vi "Synchronizator_DSBSC.vi"(8 "Czestotliwosc_probkowania":dbl, 9 "Czas":dbl, 10 "Czestotliwosc_sygnalu_nosnego":dbl, 11 "Sygnal_zmodulowany":dbl[](array[numeric])) -> (3 "Przesuniecie_fazowe":dbl)   [LabVIEW 2020]
doc: "VI zwraca przesuniecie fazowe, o ktore nalezy skorygowac generowany sygnal nosny."
uses:
  Kontrolki/Parametry_cosinusa.ctl
  <vilib>/Analysis/3filter.llb/Butterworth Filter (DBL).vi
  <vilib>/Analysis/NI_AALBase.lvlib
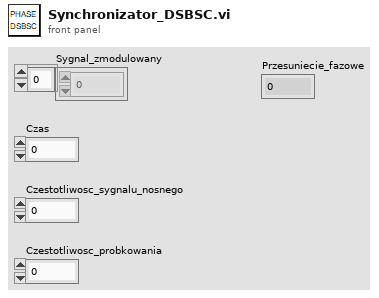
[diagram p1: front panel]
types:
  T1 = typedef "Parametry_cosinusa.ctl" = cluster{"Amplituda [V]":dbl, "Czestotliwosc [Hz] ":dbl, "Faza [rad]":dbl}
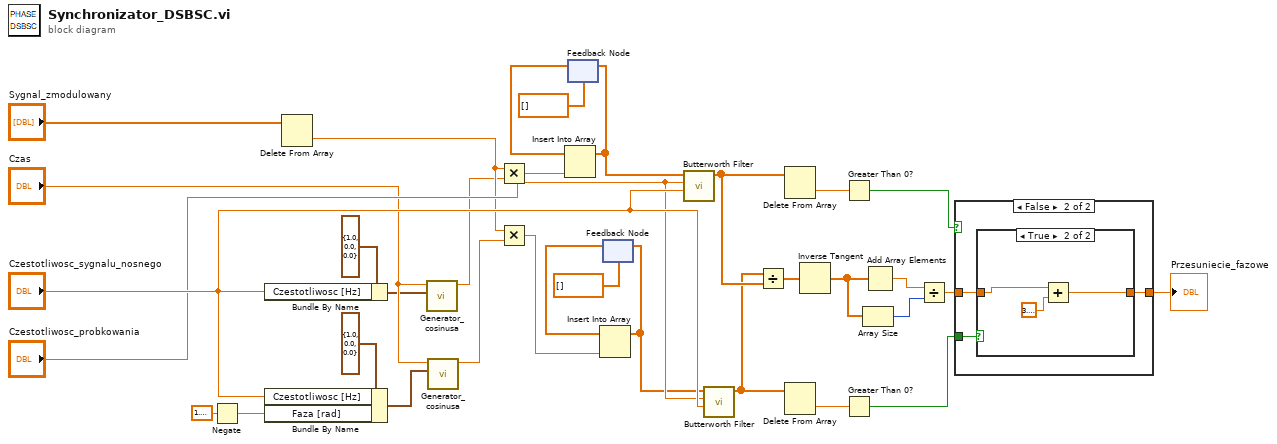
[diagram p0: block diagram]
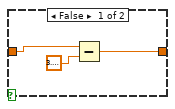
[diagram p4: hidden frame]
diagram:
  n1 = Negate(x=1.5707963267948966) -> (-x=w15:dbl)
  n2 = Bundle By Name(cluster=T1 {"Amplituda [V]"=1.0, "Czestotliwosc [Hz] "=0.0, "Faza [rad]"=0.0} ("Parametry_sygnalu_nosnego"), "Czestotliwosc [Hz]"="Czestotliwosc_sygnalu_nosnego") -> (w11:T1)
  n3 = Bundle By Name(cluster=T1 {"Amplituda [V]"=1.0, "Czestotliwosc [Hz] "=0.0, "Faza [rad]"=0.0} ("Parametry_sygnalu_nosnego"), "Czestotliwosc [Hz]"="Czestotliwosc_sygnalu_nosnego", "Faza [rad]"=w15) -> (w16:T1)
  n4 = Delete From Array(array="Sygnal_zmodulowany") -> (deleted portion=w19:dbl)  [unwired: 2 in, 1 out]
  n5 = call "Generator_cosinusa.vi"("Parametry_cosinusa"=w11, "Czas"="Czas") -> ("A cos(2pift + phi)"=w12:dbl)  [unwired: 9 in]
  n6 = call "Generator_cosinusa.vi"("Parametry_cosinusa"=w16, "Czas"="Czas") -> ("A cos(2pift + phi)"=w18:dbl)  [unwired: 9 in]
  n7 = Multiply(x=w19, y=w12) -> (x*y=w20:dbl)
  n8 = Multiply(x=w19, y=w18) -> (x*y=w27:dbl)
  n9 = feedback #1(dbl[] []) -> (w22:dbl[])
  n10 = Insert Into Array(array=w22, new element=w20) -> (w23:dbl[])  [unwired: 1 in]
  n11 = feedback-in #1(w23) -> ()
  n12 = feedback #2(dbl[] []) -> (w25:dbl[])
  n13 = Insert Into Array(array=w25, new element=w27) -> (w24:dbl[])  [unwired: 1 in]
  n14 = feedback-in #2(w24) -> ()
  n15 = call-poly <vilib>:"Butterworth Filter.vi"("high cutoff freq: fh"="Czestotliwosc_sygnalu_nosnego", "sampling freq: fs"="Czestotliwosc_probkowania", "X"=w23) -> ("Filtered X"=w8:dbl[])  [unwired: 5 in, 1 out]
  n16 = call-poly <vilib>:"Butterworth Filter.vi"("high cutoff freq: fh"="Czestotliwosc_sygnalu_nosnego", "sampling freq: fs"="Czestotliwosc_probkowania", "X"=w24) -> ("Filtered X"=w5:dbl[])  [unwired: 5 in, 1 out]
  n17 = Divide(x=w5, y=w8) -> (x/y=w30:dbl[])
  n18 = Delete From Array(array=w8) -> (deleted portion=w7:dbl)  [unwired: 2 in, 1 out]
  n19 = Delete From Array(array=w5) -> (deleted portion=w6:dbl)  [unwired: 2 in, 1 out]
  n20 = Inverse Tangent(1:w30) -> (0:w32:dbl[])
  n21 = Greater Than 0?(x=w7) -> (x > 0?=w3:bool)
  n22 = Greater Than 0?(x=w6) -> (x > 0?=w2:bool)
  n23 = Array Size(array=w32) -> (size(s)=w33:i32)
  n24 = Add Array Elements(numeric array=w32) -> (sum=w31:dbl)
  n25 = Divide(x=w31, y=w33) -> (x/y=w4:dbl)
  n26 = case shown="False" w3 {
    tunnel: w4 -> [w36 w41]
    tunnel: w2 -> [w35 w40]
    tunnel: [w34 w39] -> w1
    frame True {
      n27 = case shown="True" w35 {
        tunnel: w36 -> [w37 w38]
        tunnel: [w37 w38] -> w34
        frame False {
        }
        frame True {
        }
      }
    }
    frame False {
      n28 = case shown="True" w40 {
        tunnel: w41 -> [w43 w46]
        tunnel: [w44 w47] -> w39
        frame False {
          n29 = Subtract(x=w43, y=3.141592653589793) -> (x-y=w44:dbl)
        }
        frame True {
          n30 = Add(x=w46, y=3.141592653589793) -> (x+y=w47:dbl)
        }
      }
    }
  }
  "Przesuniecie_fazowe" <- w1
